vi "MeanImage_NoZeros.vi"(7 "Image IN":sgl[][](array[numeric]), 13 "STDev Factor":dbl format="%#_13g") -> (8 "No Zero Mean":dbl format="%0.2f")   [LabVIEW 2014]
uses:
  <vilib>/Analysis/baseanly.llb/Mean (DBL).vi
  <vilib>/Analysis/NI_AALBase.lvlib
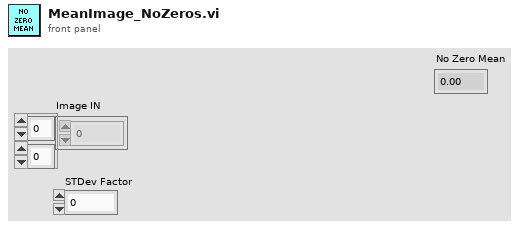
[diagram p1: front panel]
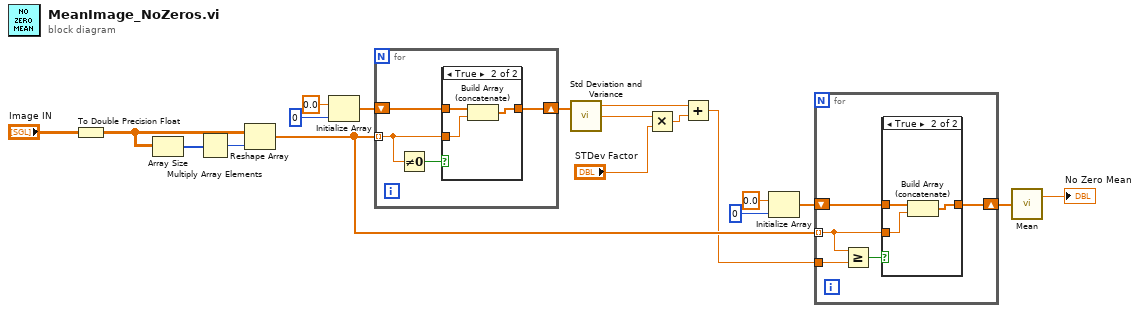
[diagram p0: block diagram]
diagram:
  n1 = To Double Precision Float(number="Image IN") -> (double precision float=w9:dbl[][])
  n2 = Array Size(array=w9) -> (size(s)=w19:i32[])
  n3 = Multiply Array Elements(1:w19) -> (0:w18:i32)
  n4 = Reshape Array(w9, w18) -> (w4:dbl[])
  n5 = Initialize Array(0.0 ("element"), 0 ("dimension size")) -> (w15:dbl[])
  n6 = for {
    tunnel: w4 -> [w21] mode=indexing
    shift-right: [w20] -> w8
    shift-left: w15 -> [w22]
    n7 = Not Equal To 0?(x=w21) -> (x != 0?=w23:bool)
    n8 = case shown="True" w23 {
      tunnel: w22 -> [w24 w27]
      tunnel: w21 -> [_ w26]
      tunnel: [w24 w25] -> w20
      frame False {
      }
      frame True {
        n9 = Build Array (concatenate)(w27, w26) -> (w25:dbl[])
      }
    }
  }
  n10 = call <vilib>:"Std Deviation and Variance.vi"("X"=w8) -> ("mean"=w11:dbl, "standard deviation"=w13:dbl)  [unwired: 1 in, 1 out]
  n11 = Multiply(x=w13, y="STDev Factor") -> (x*y=w10:dbl)
  n12 = Add(x=w11, y=w10) -> (x+y=w3:dbl)
  n13 = Initialize Array(0.0 ("element"), 0 ("dimension size")) -> (w7:dbl[])
  n14 = for {
    tunnel: w4 -> [w30] mode=indexing
    shift-right: [w31] -> w2
    shift-left: w7 -> [w32]
    tunnel: w3 -> [w28]
    n15 = Greater Or Equal?(x=w30, y=w28) -> (x >= y?=w29:bool)
    n16 = case shown="True" w29 {
      tunnel: w32 -> [w33 w36]
      tunnel: w30 -> [_ w35]
      tunnel: [w33 w34] -> w31
      frame False {
      }
      frame True {
        n17 = Build Array (concatenate)(w36, w35) -> (w34:dbl[])
      }
    }
  }
  n18 = call-poly <vilib>:"Mean.vi"("X"=w2) -> ("mean"=→"No Zero Mean":dbl)  [unwired: 1 out]
